vi "Add Tx UDP Status Section.vi"(8 "error in":errorcluster, 11 "Tx UDP ref":T1 format="%.0x") -> (0 "error out":errorcluster, 1 "Tx UDP status channel refs":T1[](array[typedef]) format="%.0x", 2 "Tx UDP status section ref out":T1 format="%.0x", 3 "Tx UDP ref out":T1 format="%.0x")   [LabVIEW 2020, in "AIM ARINC 664 Scripting.lvlib"]
uses:
  AIM ARINC 664 Scripting.lvlib
  <vilib>/NI VeriStand/Custom Device API/Custom Device Item Ref.ctl
  Constants.vi
  <vilib>/Utility/Data Type/NI_Data Type.lvlib
  Shared/Tx Generic Queue Status Enum.ctl
  <vilib>/NI VeriStand/Custom Device API/Custom Device API.lvlib
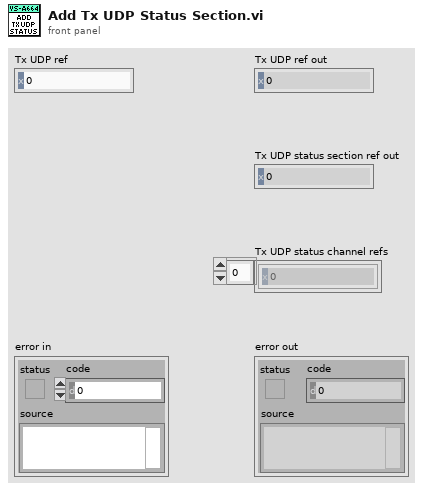
[diagram p1: front panel]
types:
  T1 = typedef "Custom Device API.lvlib/Custom Device Item Ref.ctl" = u64
  T2 = typedef "Tx Generic Queue Status Enum.ctl" = enum16{"FDX_QUE_EMPTY", "FDX_QUE_FILLED", "FDX_QUE_FULL", "FDX_QUE_SENT", "FDX_QUE_CYCL_RUN", "FDX_QUE_CYCL_SENT"}
  T3 = cluster{"Rx UDP Status":string, "enum names":string[], "Values":dbl[]}
  T4 = cluster{"Rx UDP Status":string, "enum names":string[], "Values":dbl[]}[]
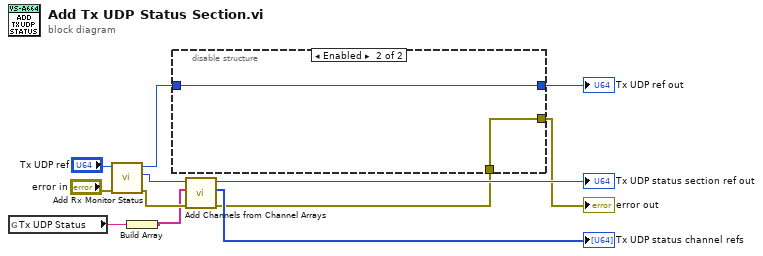
[diagram p0: block diagram]
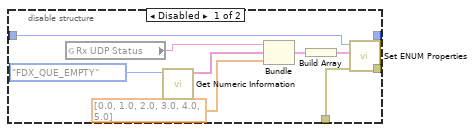
[diagram p2: hidden frame]
diagram:
  n1 = global read "Constants.vi" "Tx UDP Status"() -> (w1:string)
  n2 = call "Add Rx Monitor Status.vi"("error in (no error)"="error in", "Rx monitor ref in"="Tx UDP ref") -> ("error out"=w5:errorcluster, "Rx monitor status ref out"=w4:T1, "Rx monitor ref out"=w3:T1)  [unwired: 7 in]
  n3 = Build Array(w1) -> (w2:string[])
  n4 = call "Add Channels from Channel Arrays.vi"("error in"=w5, "channel array"=w2, "section ref in"=w4) -> ("error out"=w10:errorcluster, "channel refs"=→"Tx UDP status channel refs":T1[], "section ref out"=→"Tx UDP status section ref out":T1)  [unwired: 6 in]
  n5 = disable-structure shown="Enabled" {
    disable-tunnel: w10 -> [w17 w23]
    disable-tunnel: [w16 w23] -> w9
    disable-tunnel: [w15 w24] -> w8
    disable-tunnel: w3 -> [w14 w24]
    frame Disabled {
      n6 = global read "Constants.vi" "Rx UDP Status"() -> (w13:string)
      n7 = call <vilib>:"Get Numeric Information.vi"("variant"=Tx_Generic_Queue_Status_Enum."FDX_QUE_EMPTY") -> ("enum names"=w20:string[])  [unwired: 7 in, 3 out]
      n8 = Bundle("Rx UDP Status"=w13, "enum names"=w20, "Values"=dbl[] [0.0, 1.0, 2.0, 3.0, 4.0, 5.0]) -> (w18:T3)  [unwired: 1 in]
      n9 = Build Array(w18) -> (w21:T4)
      n10 = call "Set ENUM Properties.vi"("error in"=w17, "enum to be changes"=w21, "parent ref in"=w14) -> ("error out"=w16:errorcluster, "parent ref out"=w15:T1)  [unwired: 7 in]
    }
    frame Enabled {
    }
  }
  "Tx UDP ref out" <- w8
  "error out" <- w9
